vi "Start.vi"(8 "error in (no error)":errorcluster, 10 "Message in":refnum<class "StartMessage.lvclass">, 11 "Retiga in":refnum<class "Retiga.lvclass">) -> (0 "error out":errorcluster, 3 "Retiga out":refnum<class "Retiga.lvclass">)   [LabVIEW 2012, in "Retiga.lvclass"]
doc: "This member function is called when the statemachine in the run.vi receives an 'start' command. It relays the message to all observers of the component.\n\nOverride this member function in your derived class if you need additional start functionality (but don't forget to call the parent method)."
uses:
  Retiga.lvclass
  <vilib>/Distrio/Murmex/StartMessage/StartMessage.lvclass
  <vilib>/Distrio/Murmex/Murmex/Murmex.lvclass
  <vilib>/Distrio/Murmex/ProceedMessage/ProceedMessage.lvclass
panel:
  # "This member function is called when the statemachine in the run.vi receives an 'start' command. It relays the message to all observers of the component.\n\nOverride this member function in your derived class if you need additional start functionality (but don't forget to call the parent method)."
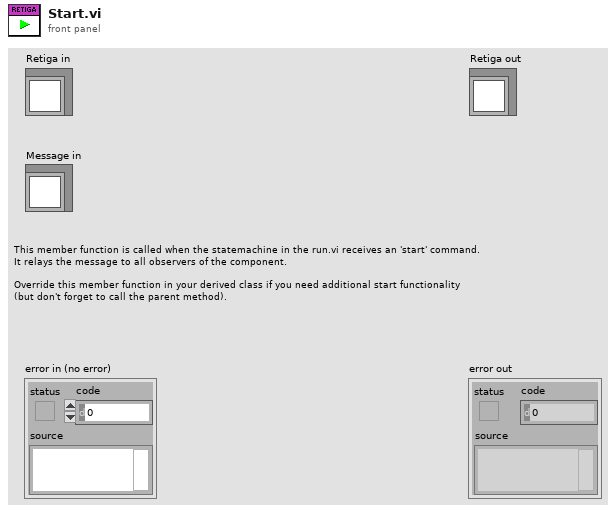
[diagram p1: front panel]
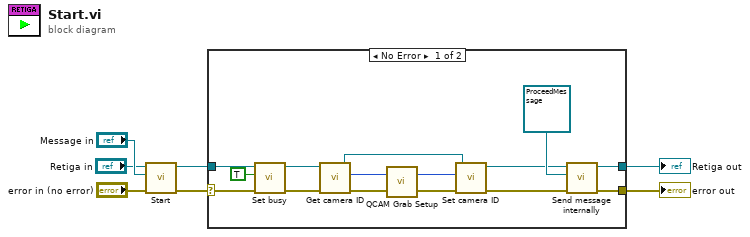
[diagram p0: block diagram]
diagram:
  n1 = call-parent "Start.vi"("error in (no error)"="error in (no error)", "Message in"="Message in", "Murmex in"="Retiga in") -> ("error out"=w4:errorcluster, "Murmex out"=w1:refnum<class "Retiga.lvclass">)  [unwired: 7 in]
  n2 = case shown="No Error" w4 {
    selector: w4 -> [w22 w24]
    tunnel: [w8 w24] -> w3
    tunnel: [w9 w23] -> w2
    tunnel: w1 -> [w21 w23]
    frame No Error {
      n3 = call-dynamic "Set busy.vi"("error in (no error)"=w22, "busy?"=TRUE, "Retiga in"=w21) -> ("error out"=w18:errorcluster, "Retiga out"=w19:refnum<class "Retiga.lvclass">)  [unwired: 7 in]
      n4 = call-dynamic "Get camera ID.vi"("error in (no error)"=w18, "Retiga in"=w19) -> ("error out"=w17:errorcluster, "camera ID"=w16:u32, "Retiga out"=w13:refnum<class "Retiga.lvclass">)  [unwired: 7 in]
      n5 = call <userlib>:"QCAM Grab Setup.vi"("error in (no error)"=w17, "cameraId"=w16) -> ("error out"=w14:errorcluster, "cameraId out"=w15:u32)
      n6 = call-dynamic "Set camera ID.vi"("error in (no error)"=w14, "camera ID"=w15, "Retiga in"=w13) -> ("error out"=w11:errorcluster, "Retiga out"=w10:refnum<class "Retiga.lvclass">)  [unwired: 7 in]
      n7 = call <vilib>:"Send message internally.vi"("error in (no error)"=w11, "Message"=refnum<class "ProceedMessage.lvclass"> refnum ("ProceedMessage"), "Murmex in"=w10) -> ("error out"=w8:errorcluster, "Murmex out"=w9:refnum<class "Retiga.lvclass">)  [unwired: 7 in]
    }
    frame Error {
    }
  }
  "error out" <- w3
  "Retiga out" <- w2
